vi "F Dwf Digital Out Counter Init Set.vi"(7 "v":u32, 8 "error in (no error)":errorcluster, 9 "fHigh":i32, 10 "idxChannel":i32, 11 "hdwf":i32) -> (0 "error out":errorcluster, 3 "function return":i32)   [LabVIEW 2019, in "Olasdwf.lvlib"]
doc: "DWFAPI int FDwfDigitalOutCounterInitSet(HDWF hdwf, int idxChannel, int fHigh, unsigned int v);"
uses:
  Olasdwf.lvlib
  Windows/System32/dwf.dll
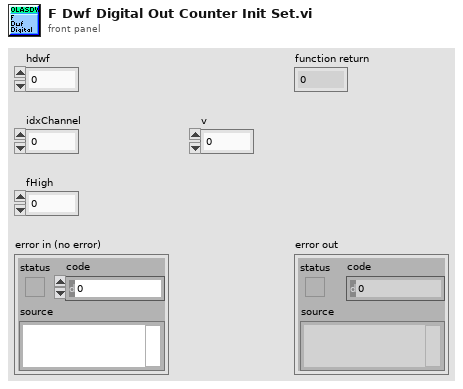
[diagram p1: front panel]
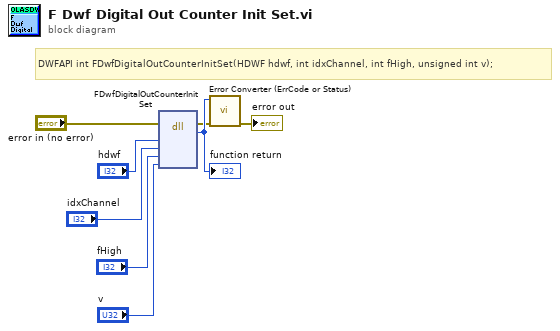
[diagram p0: block diagram]
diagram:
  # "DWFAPI int FDwfDigitalOutCounterInitSet(HDWF hdwf, int idxChannel, int fHigh, unsigned int v);"
  n1 = dll-call lib="C:/Windows/System32/dwf.*" fn="FDwfDigitalOutCounterInitSet"(error in="error in (no error)", "hdwf"="hdwf", "idxChannel"="idxChannel", "fHigh"="fHigh", "v"="v") -> (error out=w2:errorcluster, w8:i32)  [unwired: 6 in, 1 out]
  "function return" <- w8
  n2 = call "Error Converter (ErrCode or Status).vi"("error in (no error)"=w2, "error code"=w8) -> ("error out"=→"error out":errorcluster)  [unwired: 9 in]
